vi "Channel Level.vi"(8 "error in (no error)":errorcluster, 11 "Node Ptr":T1 format="%.0x") -> (0 "error out":errorcluster)   [LabVIEW 2023, in "Embedded TDMS Logger System Explorer.lvlib"]
uses:
  Embedded TDMS Logger System Explorer.lvlib
  <vilib>/NI VeriStand/Custom Device API/Custom Device Item Ref.ctl
  Shared/Meta Data Item.ctl
  <vilib>/NI VeriStand/Custom Device API/Get Item Property (Variant).vi
  <vilib>/NI VeriStand/Custom Device API/Set Item Property (Variant).vi
  <vilib>/NI VeriStand/Custom Device API/Custom Device API.lvlib
  Shared/Embedded TDMS Logger Shared.lvlib
panel:
  in  "Channel Level Meta Data":string[][](table)
  in  "Specific Header":cluster{"Section Name":string}={"Section Name"="Specific Page Settings"}
  in  "General Header":cluster{"Section Name":string}={"Section Name"="General Page Settings"}
  in  "Description":string
  in  "Channel Name":string
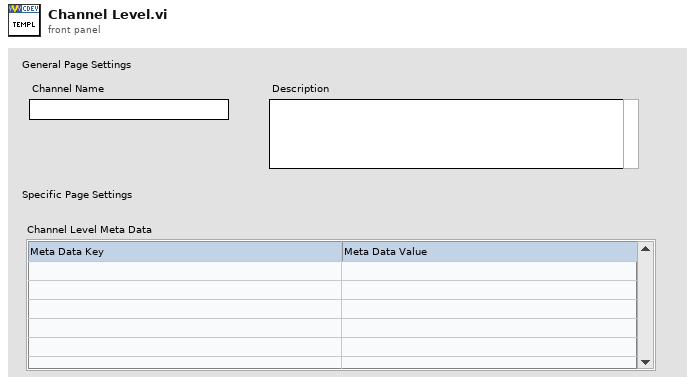
[diagram p1: front panel]
types:
  T1 = typedef "Custom Device API.lvlib/Custom Device Item Ref.ctl" = u64
  T2 = typedef "Embedded TDMS Logger Shared.lvlib/Meta Data Item.ctl" = cluster{"Key":string, "Value":string}
  T3 = typedef "Custom Device API.lvlib/Custom Device Item Info.ctl" = cluster{"Name":string, "Is Channel":bool, "GUID":string, "Is Waveform":bool}
  T4 = typedef "Custom Device API.lvlib/Custom Device Commands.ctl" = enum16{"Default", "Item renamed", "Shutdown", "Dynamic button pressed"}
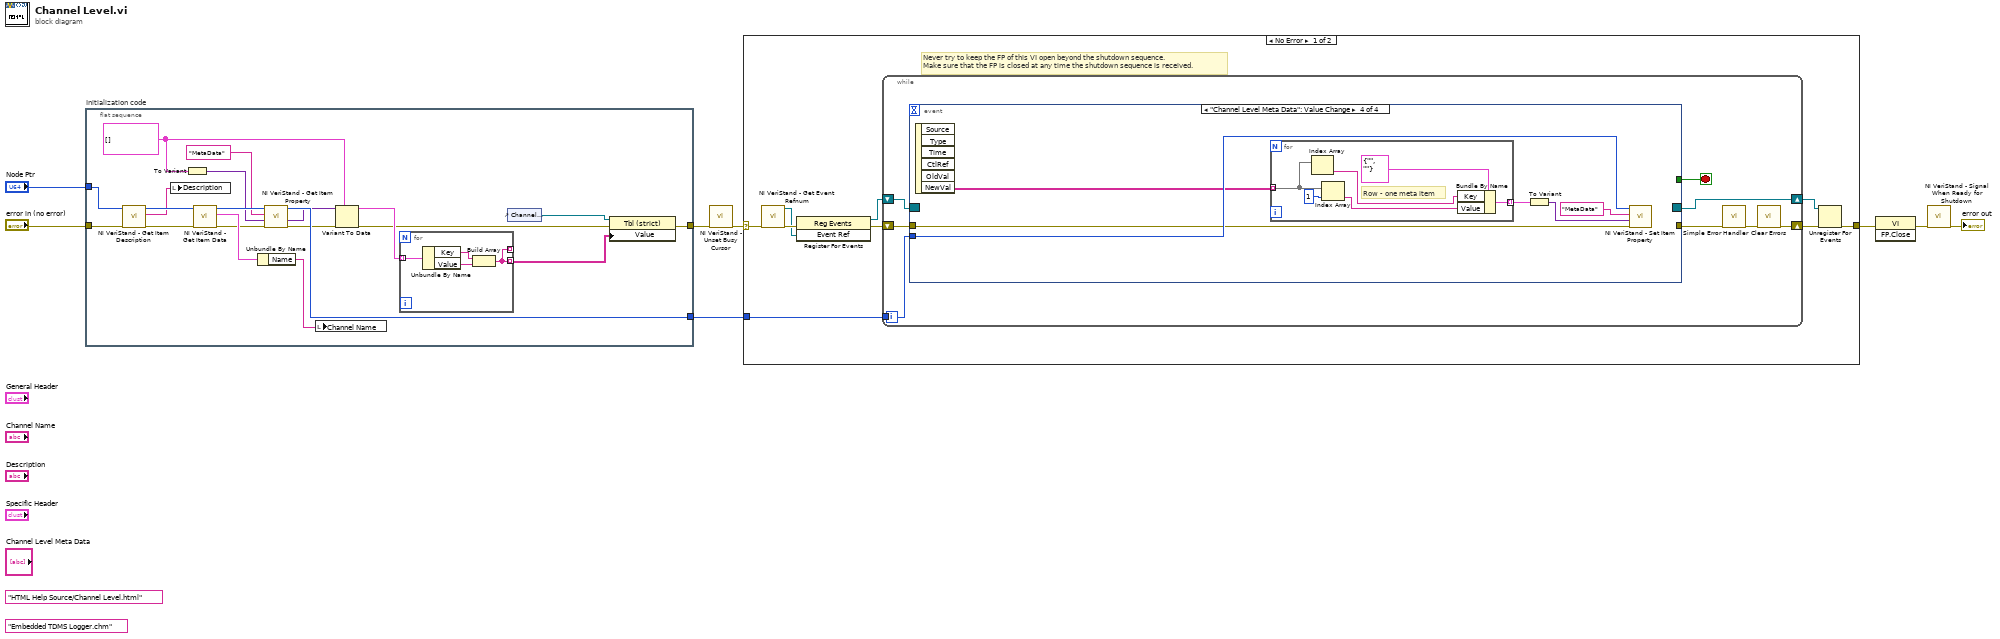
[diagram p0: block diagram]
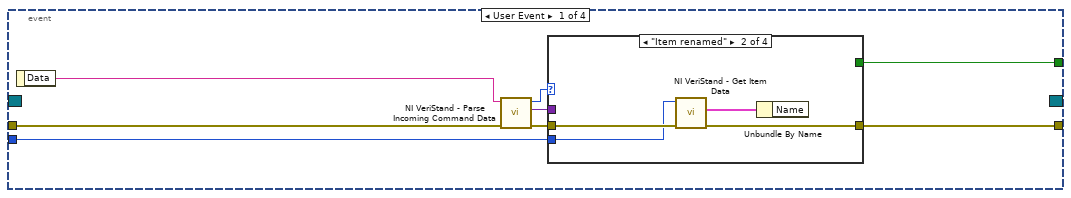
[diagram p2: hidden frame]
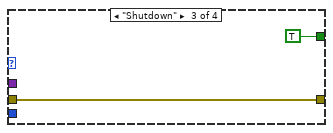
[diagram p4: hidden frame]
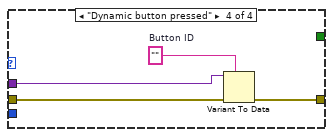
[diagram p5: hidden frame]
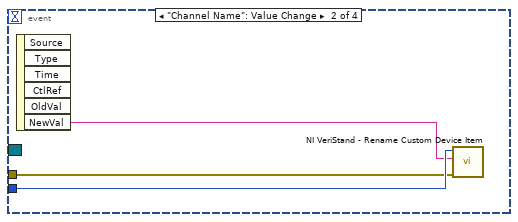
[diagram p6: hidden frame]
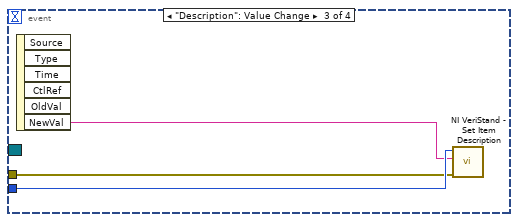
[diagram p7: hidden frame]
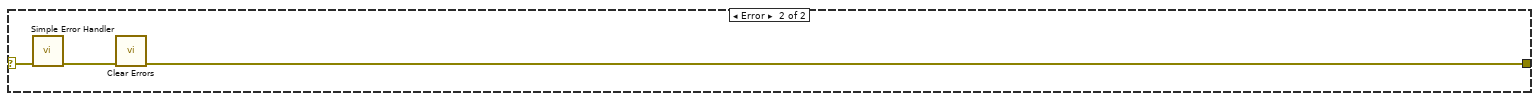
[diagram p8: hidden frame]
diagram:
  (unwired) "HTML Help Source/Channel Level.html" ("CD_CHM_Section")
  (unwired) "Embedded TDMS Logger.chm" ("CD_CHM_FileName")
  n1 = flat-sequence "Initialization code" {
    tunnel: "Node Ptr" -> [w9]
    tunnel: [w12] -> w3
    tunnel: [w20] -> w4
    tunnel: "error in (no error)" -> [w10]
    frame #0 {
      w16 = T2[] []
      n2 = call <vilib>:"NI VeriStand - Get Item Description.vi"("error in (no error)"=w10, "Item Ref in"=w9) -> ("error out"=w27:errorcluster, "Description"=w24:string, "Item Ref out"=w28:T1)  [unwired: 7 out]
      n3 = local write "Description"(w24) -> ()
      n4 = To Variant(anything=w16) -> (Variant=w19:variant)
      n5 = call <vilib>:"NI VeriStand - Get Item Data.vi"("error in (no error)"=w27, "Item Ref in"=w28) -> ("error out"=w23:errorcluster, "Item Info"=w26:T3, "Item Ref out"=w22:T1)  [unwired: 7 out]
      n6 = Unbundle By Name(w26) -> ("Name"=w25:string)
      n7 = call-poly <vilib>:"NI VeriStand - Get Item Property.vi"("error in (no error)"=w23, "Default Value"=w19, "Property Name"="MetaData", "Item Ref in"=w22) -> ("error out"=w18:errorcluster, "Value"=w17:variant, "Item Ref out"=w20:T1)  [unwired: 4 in, 1 out]
      n8 = local write "Channel Name"(w25) -> ()
      n9 = Variant To Data(error in=w18, type=w16, Variant=w17) -> (data=w15:T2[], error out=w13:errorcluster)
      n10 = for {
        tunnel: w15 -> [w32] mode=indexing
        tunnel: [w29] -> _ mode=indexing
        tunnel: [w29] -> w14 mode=indexing
        n11 = Unbundle By Name(w32) -> ("Key"=w31:string, "Value"=w30:string)
        n12 = Build Array(w31, w30) -> (w29:string[])
      }
      n13 = control-ref of="Channel Level Meta Data"() -> (w11:refnum<vi>)
      n14 = property class="Tbl (strict)"(reference=w11, error in=w13, "Value"=w14) -> (error out=w12:errorcluster)  [unwired: 1 out]
    }
  }
  n15 = call <vilib>:"NI VeriStand - Unset Busy Cursor.vi"("error in (no error)"=w3) -> ("error out"=w5:errorcluster)  [unwired: 10 out]
  n16 = case shown="No Error" w5 {
    selector: w5 -> [w33 w89]
    tunnel: [w38 w87] -> w8
    tunnel: w4 -> [w34 _]
    frame No Error {
      # "Never try to keep the FP of this VI open beyond the shutdown sequence.\nMake sure that the FP is closed at any time the shutdown sequence is received."
      n17 = call <vilib>:"NI VeriStand - Get Event Refnum.vi"("error in (no error)"=w33) -> ("error out"=w41:errorcluster, "Event Ref"=w37:refnum<user-event>)  [unwired: 9 out]
      n18 = register-events(error in=w41, w37) -> (reference out=w35:refnum<event-registration>, error out=w36:errorcluster)  [unwired: 1 in]
      n19 = while {
        tunnel: w34 -> [w45]
        shift-right: [w42] -> w39
        shift-left: w36 -> [w48]
        shift-right: [w49] -> w40
        shift-left: w35 -> [w47]
        stop <- w46 stop-if-true
        n20 = event shown="[3] \"Channel Level Meta Data\": Value Change" {
          selector: w47 -> [_ _ _ _]
          dyn-events: [_ _ _ _] -> w49
          timeout: _ -> [_ _ _ _]
          tunnel: w48 -> [w57 w69 w73 w75]
          tunnel: [w53 _ _ _] -> w46
          tunnel: [w52 _ _ _] -> w44
          tunnel: w45 -> [w51 w71 w74 w77]
          event User Event {
            n21 = event-data() -> ("Data"=w56:string)  [unwired: 1 out]
            n22 = call <vilib>:"NI VeriStand - Parse Incoming Command Data.vi"("error in (no error)"=w57, "Incoming data"=w56) -> ("error out"=w55:errorcluster, "Outgoing data"=w50:variant, "Action"=w54:T4)  [unwired: 7 out]
            n23 = case shown="\"Item renamed\"" w54 {
              tunnel: w55 -> [w58 w62 w63 w68]
              tunnel: [_ _ TRUE _] -> w53
              tunnel: [w58 w59 w63 w65] -> w52
              tunnel: w51 -> [_ w61 _ _]
              tunnel: w50 -> [_ _ _ w67]
              frame "Default", Default {
              }
              frame "Item renamed" {
                n24 = call <vilib>:"NI VeriStand - Get Item Data.vi"("error in (no error)"=w62, "Item Ref in"=w61) -> ("error out"=w59:errorcluster, "Item Info"=w60:T3)  [unwired: 8 out]
                n25 = Unbundle By Name(w60) -> ()  [unwired: 1 out]
              }
              frame "Shutdown" {
              }
              frame "Dynamic button pressed" {
                w66 = ""  # Button ID
                n26 = Variant To Data(error in=w68, type=w66, Variant=w67) -> (error out=w65:errorcluster)  [unwired: 1 out]
              }
            }
          }
          event "Channel Name": Value Change {
            n27 = event-data() -> ("NewVal"=w70:string)  [unwired: 6 out]
            n28 = call <vilib>:"NI VeriStand - Rename Custom Device Item.vi"("error in (no error)"=w69, "New Name"=w70, "Item Ref in"=w71) -> ()  [unwired: 6 in, 3 out]
          }
          event "Description": Value Change {
            n29 = event-data() -> ("NewVal"=w72:string)  [unwired: 6 out]
            n30 = call <vilib>:"NI VeriStand - Set Item Description.vi"("error in (no error)"=w73, "Description"=w72, "Item Ref in"=w74) -> ()  [unwired: 6 in, 3 out]
          }
          event "Channel Level Meta Data": Value Change {
            n31 = event-data() -> ("NewVal"=w76:string[][])  [unwired: 6 out]
            n32 = for {
              tunnel: w76 -> [w85] mode=indexing
              tunnel: [w81] -> w80 mode=indexing
              # "Row - one meta item"
              n33 = Index Array(array=w85) -> (element=w82:string)  [unwired: 1 in]
              n34 = Index Array(array=w85, index=1) -> (element=w83:string)
              n35 = Bundle By Name(cluster=T2 {"Key"="", "Value"=""} ("Meta Data"), "Key"=w82, "Value"=w83) -> (w81:T2)
            }
            n36 = To Variant(anything=w80) -> (Variant=w79:variant)
            n37 = call-poly <vilib>:"NI VeriStand - Set Item Property.vi"("error in (no error)"=w75, "Value"=w79, "Property Name"="MetaData", "Item Ref in"=w77) -> ()  [unwired: 5 in, 3 out]
          }
        }
        n38 = call <vilib>:"Simple Error Handler.vi"("error in (no error)"=w44) -> ("error out"=w43:errorcluster)  [unwired: 1 in, 7 out]
        n39 = call <vilib>:"Clear Errors.vi"("error in (no error)"=w43) -> ("error out"=w42:errorcluster)  [unwired: 1 in, 5 out]
      }
      n40 = Unregister For Events(event registration refnum=w40, error in=w39) -> (error out=w38:errorcluster)
    }
    frame Error {
      n41 = call <vilib>:"Simple Error Handler.vi"("error in (no error)"=w89) -> ("error out"=w88:errorcluster)  [unwired: 1 in, 7 out]
      n42 = call <vilib>:"Clear Errors.vi"("error in (no error)"=w88) -> ("error out"=w87:errorcluster)  [unwired: 1 in, 5 out]
    }
  }
  n43 = invoke class="VI" method="FP.Close"(error in=w8) -> (error out=w7:errorcluster)  [unwired: 2 in, 2 out]
  n44 = call <vilib>:"NI VeriStand - Signal When Ready for Shutdown.vi"("error in (no error)"=w7) -> ("error out"=→"error out":errorcluster)  [unwired: 10 out]
